vi "RUSHLights.vi"(8 "In Time":dbl, 9 "Input":bool, 10 "SP 1":bool, 11 "Lock On Ligts":dbl) -> (1 "Out Time":dbl, 2 "Output":bool, 3 "RelayValue":T1)   [LabVIEW 2011]
uses:
  <vilib>/Rock Robotics/WPI/Relay/WPI_RelayValue.ctl
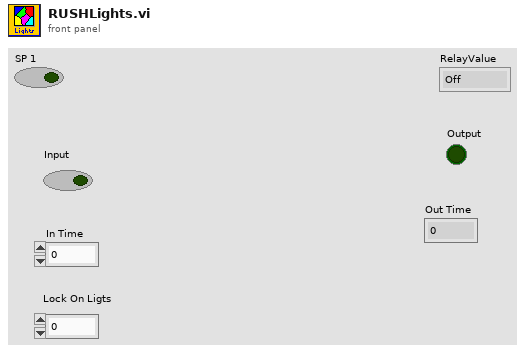
[diagram p1: front panel]
types:
  T1 = typedef "WPI_RelayValue.ctl" = enum16{"Off", "On", "Forward", "Reverse"}
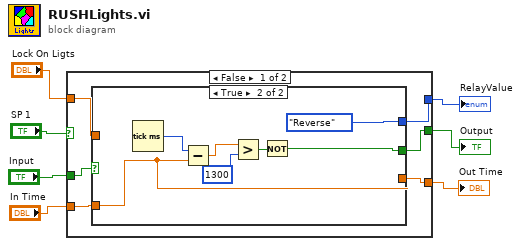
[diagram p0: block diagram]
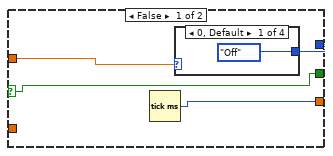
[diagram p2: hidden frame]
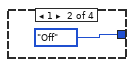
[diagram p3: hidden frame]
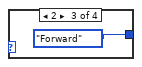
[diagram p4: hidden frame]
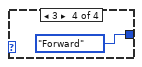
[diagram p5: hidden frame]
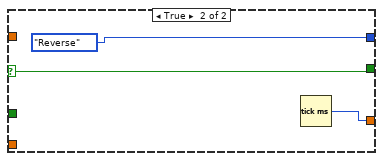
[diagram p6: hidden frame]
diagram:
  n1 = case shown="False" "SP 1" {
    selector: "SP 1" -> [_ w29]
    tunnel: [w13 WPI_RelayValue."Reverse" ("RelayValue")] -> w7
    tunnel: [w11 w30] -> w2
    tunnel: "In Time" -> [w12 _]
    tunnel: "Input" -> [w10 _]
    tunnel: [w9 w29] -> w4
    tunnel: "Lock On Ligts" -> [w8 _]
    frame False {
      n2 = case shown="True" w10 {
        selector: w10 -> [w15 _]
        tunnel: [w17 WPI_RelayValue."Reverse" ("RelayValue")] -> w13
        tunnel: w12 -> [_ w23]
        tunnel: [w16 w23] -> w11
        tunnel: [w15 w22] -> w9
        tunnel: w8 -> [w14 _]
        frame False {
          n3 = Tick Count (ms)() -> (millisecond timer value=w16:u32)
          n4 = case shown="0, Default" w14 {
            tunnel: [WPI_RelayValue."Off" ("RelayValue") WPI_RelayValue."Off" ("RelayValue") WPI_RelayValue."Forward" ("RelayValue") WPI_RelayValue."Forward" ("RelayValue")] -> w17
            frame 0, Default {
            }
            frame 1 {
            }
            frame 2 {
            }
            frame 3 {
            }
          }
        }
        frame True {
          n5 = Tick Count (ms)() -> (millisecond timer value=w27:u32)
          n6 = Subtract(x=w27, y=w23) -> (x-y=w26:dbl)
          n7 = Greater?(x=w26, y=u32 1300) -> (0:w24:bool)
          n8 = Not(x=w24) -> (.not. x?=w22:bool)
        }
      }
    }
    frame True {
      n9 = Tick Count (ms)() -> (millisecond timer value=w30:u32)
    }
  }
  "RelayValue" <- w7
  "Output" <- w4
  "Out Time" <- w2
